vi "Main.vi"(11 "Module Admin":refnum<class "Delacor_lib_QMH_Module Admin.lvclass">) -> ()   [LabVIEW 2020, in "Logger.lvlib"]
doc: "This template is based off of the Queued Message Handler design pattern and the Queued Message Handler project template that ships with LabVIEW.\n\nThe main difference is that the queue is private to this module and communication between modules is performed via Broadcast and Request events.\n\nRequest events are wrapped in public API methods and are handled in the Event Handling Loop (EHL) of this VI. Any module can register for Broadcast events sent by this module. The EHL generates messages based on user interface actions.\n\nThe Message Handling Loop (MHL) processes messages generated by the EHL, or by other messages. The messages are string values, so new messages can be added easily to the Message Cases case structure in the MHL. Each message cluster can also provide an optional value for Message Data, which is a variant that can be converted to whatever message-specific data is required.\n_____\nBased on Delacor QMH Project Template 4.0.0.47.\n_____\nBased on DQMH Project Template 6.0.0.91."
uses:
  Logger.lvlib
  <vilib>/Delacor/Delacor QMH/Libraries/Module Admin_class/Delacor_lib_QMH_Module Admin.lvclass
  Module Data--cluster.ctl
  Stop Argument--cluster.ctl
  <vilib>/Delacor/Delacor QMH/Libraries/Message Queue_class/Delacor_lib_QMH_Message Queue.lvclass/Delacor_lib_QMH_Message Queue.ctl
  <vilib>/Delacor/Delacor QMH/Libraries/Module Admin_class/Delacor_lib_QMH_Module Admin.lvclass/Delacor_lib_QMH_Module Admin.ctl
  Initialize File Argument--cluster.ctl
  Initialize File (Reply Payload)--cluster.ctl
  Log Data Argument--cluster.ctl
  Stop Logging Argument--cluster.ctl
  Settings Editor/Update Application Settings (Reply Payload)--cluster.ctl
  Settings Editor/Settings--cluster.ctl
  CML Shared/Signal Type--enum.ctl
  CML Shared/Calibration Values--cluster.ctl
  <vilib>/Utility/miscctls.llb/LVPointTypeDef.ctl
  <vilib>/Delacor/Delacor QMH/Libraries/Message Queue_class/Delacor_lib_QMH_Enqueue Message (Single).vi
  <vilib>/Delacor/Delacor QMH/Libraries/Module Admin_class/Delacor_lib_QMH_Get External Launch.vi
  <vilib>/Utility/error.llb/Error Cluster From Error Code.vi
  <vilib>/ErrorRing/Error Ring.xnode
  <vilib>/Delacor/Delacor QMH/Libraries/Message Queue_class/Delacor_lib_QMH_Message Queue.lvclass
  Settings Editor/Settings Editor.lvlib
  CML Shared/CML Shared.lvlib
panel:
  out "Settings":T1
  out "error out":errorcluster
  # "This is a headless module. Show its panel to confirm that the Settings are updated correctly and other debugging tasks. Use the Settings Editor to change the settings for this module."
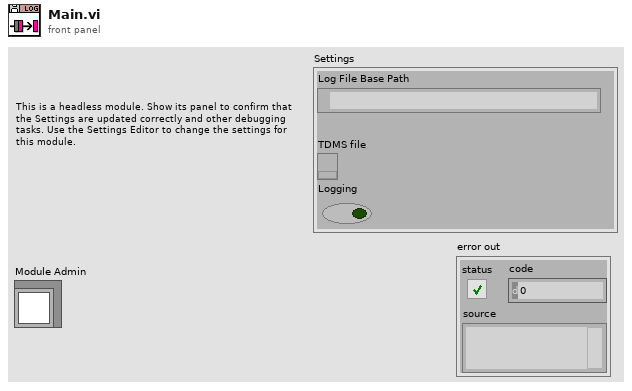
[diagram p1: front panel]
types:
  T1 = typedef "Logger.lvlib/Module Data--cluster.ctl" = cluster{"Log File Base Path":path, "TDMS file":refnum<k34>, "Logging":bool}
  T2 = typedef "Settings Editor.lvlib/Broadcast Events--cluster.ctl" = cluster{"Module Did Init":refnum<user-event>, "Status Updated":refnum<user-event>, "Error Reported":refnum<user-event>, "Module Did Stop":refnum<user-event>, "Update Module Execution Status":refnum<user-event>, "Application Settings Updated":refnum<user-event>}
  T3 = typedef "Logger.lvlib/Request Events--cluster.ctl" = cluster{"Stop Module":refnum<user-event>, "Show Panel":refnum<user-event>, "Hide Panel":refnum<user-event>, "Get Module Execution Status":refnum<user-event>, "Show Diagram":refnum<user-event>, "Stop Logging":refnum<user-event>, "Log Data":refnum<user-event>, "Initialize File":refnum<user-event>}
  T4 = enum32{"invalid lock state", "Not Locked", "Locked (No Password)", "Password-protected"}
  T5 = typedef "Logger.lvlib/Stop Argument--cluster.ctl" = cluster{"Origin":string, "Exit via Stop Module Req?":bool, "Wait for Module to stop?":bool}
  T6 = typedef "Logger.lvlib/Initialize File Argument--cluster.ctl" = cluster{"Wait Notifier":refnum<notifier>, "wait for reply":bool}
  T7 = typedef "Logger.lvlib/Log Data Argument--cluster.ctl" = cluster{"Waveforms":waveform(dbl)[]}
  T8 = typedef "Logger.lvlib/Stop Logging Argument--cluster.ctl" = cluster{"Boolean":bool}
  T9 = typedef "Settings Editor.lvlib/Update Application Settings (Reply Payload)--cluster.ctl" = cluster{"Settings":T10, "Update Settings_error":errorcluster}
  T10 = typedef "Settings Editor.lvlib/Settings--cluster.ctl" = cluster{"Signal Type":T11, "Calibration Array":T12[], "Log File Base Path":path}
  T11 = typedef "CML Shared.lvlib/Signal Type--enum.ctl" = enum16{"Sine Wave", "Square with Noise"}
  T12 = typedef "CML Shared.lvlib/Calibration Values--cluster.ctl" = cluster{"Slope":dbl, "Offset":dbl}
  T13 = typedef "LVPointTypeDef.ctl" = cluster{"Horizontal":i16, "Vertical":i16}
  T14 = enum32{"Invalid", "Standard", "Closed", "Hidden", "Minimized", "Maximized"}
  T15 = typedef "Logger.lvlib/Initialize File (Reply Payload)--cluster.ctl" = cluster{"File Path":path, "Initialize File_error":errorcluster}
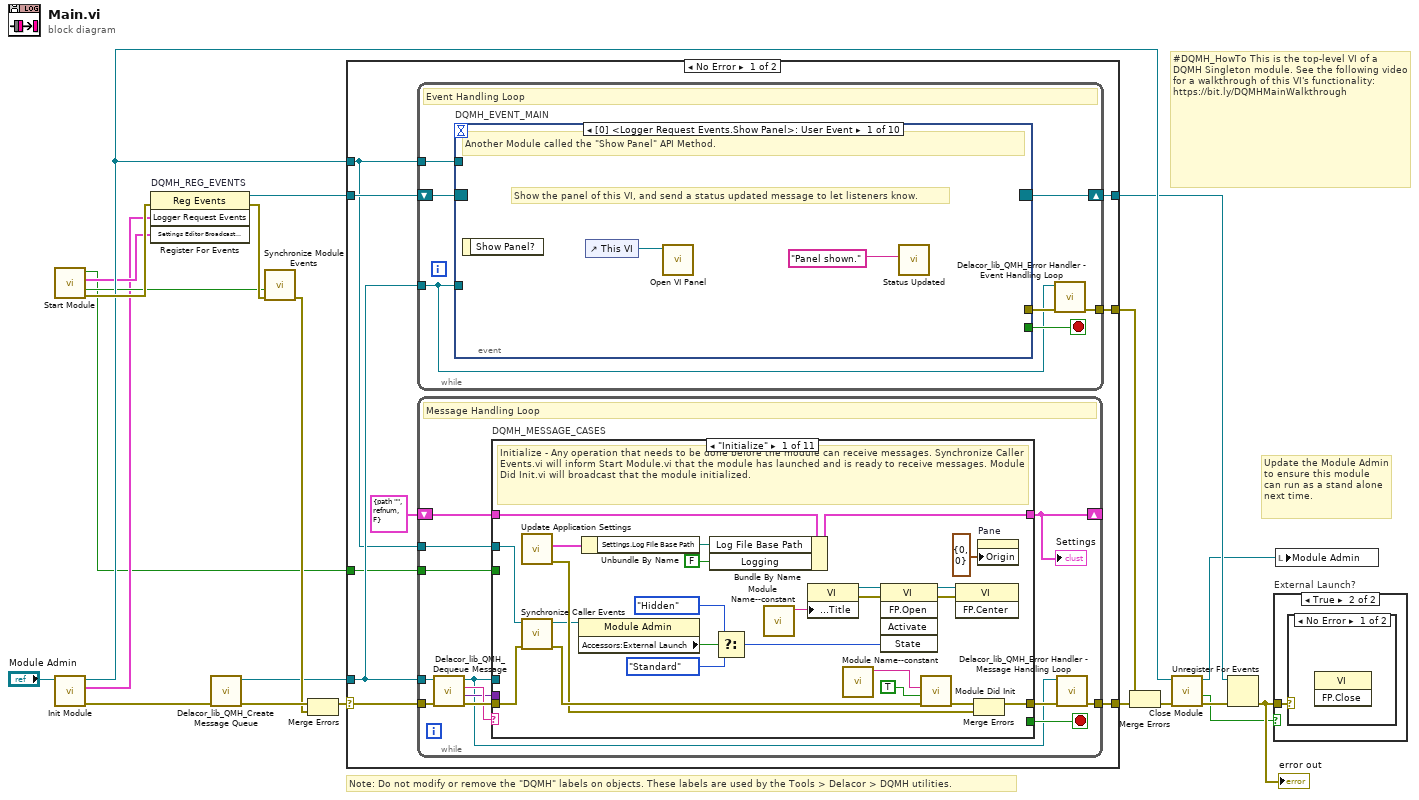
[diagram p0: block diagram]
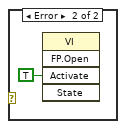
[diagram p3: hidden frame]
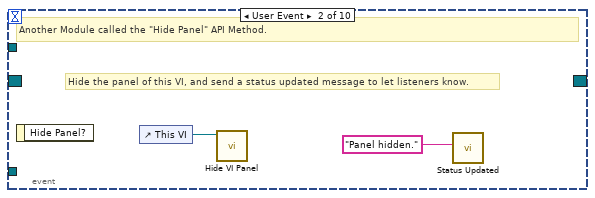
[diagram p4: hidden frame]
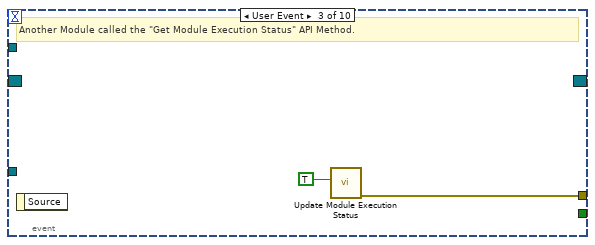
[diagram p5: hidden frame]
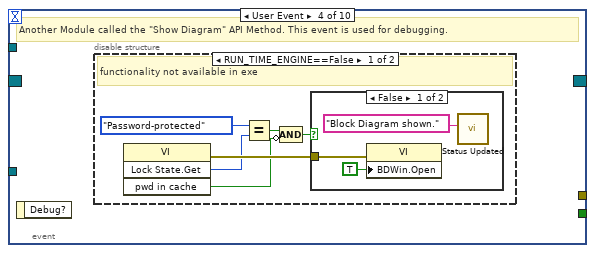
[diagram p6: hidden frame]
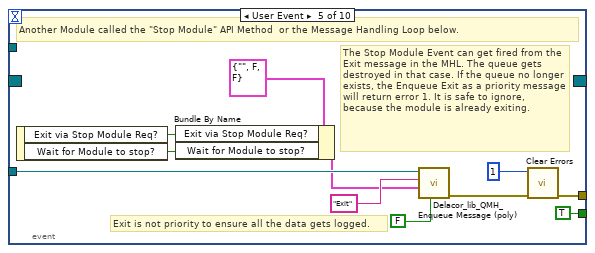
[diagram p9: hidden frame]
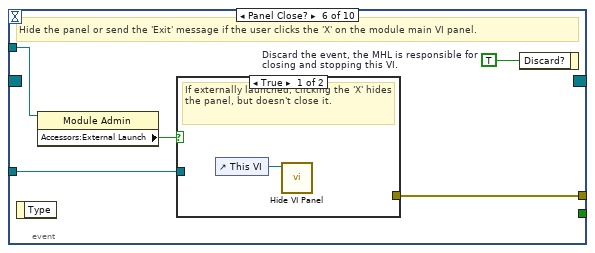
[diagram p10: hidden frame]
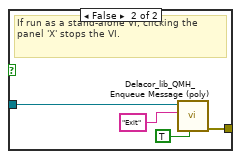
[diagram p11: hidden frame]
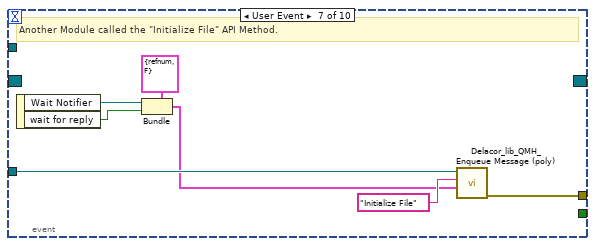
[diagram p12: hidden frame]
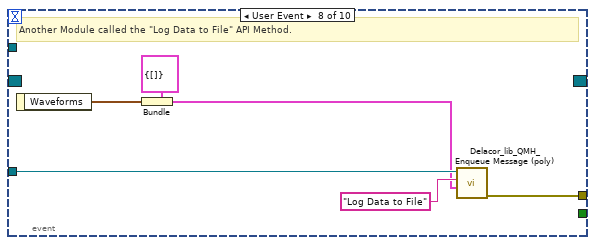
[diagram p13: hidden frame]
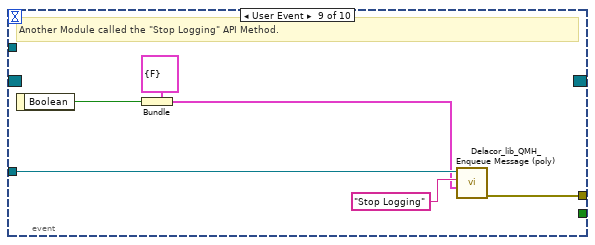
[diagram p14: hidden frame]
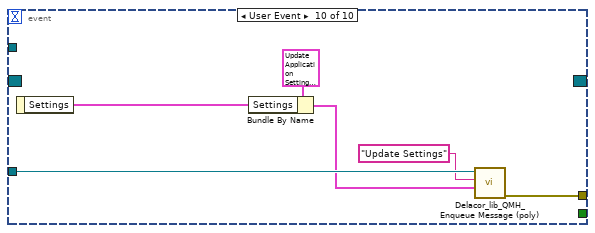
[diagram p15: hidden frame]
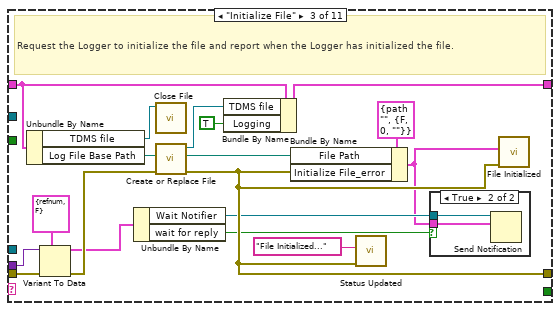
[diagram p17: hidden frame]
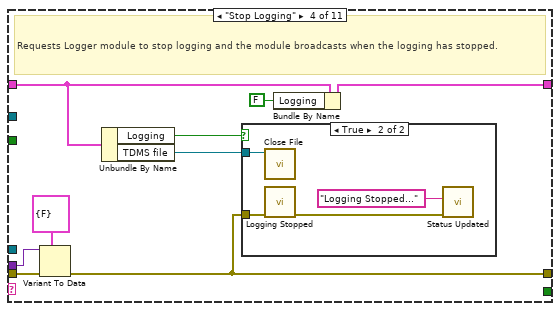
[diagram p19: hidden frame]
diagram:
  # "#DQMH_HowTo This is the top-level VI of a DQMH Singleton module. See the following video for a walkthrough of this VI's functionality: https://bit.ly/DQMHMainWalkthrough"
  # "Note: Do not modify or remove the \"DQMH\" labels on objects. These labels are used by the Tools > Delacor > DQMH utilities."
  # "Update the Module Admin to ensure this module can run as a stand alone next time."
  n1 = call "Start Module.vi"() -> ("error out"=w14:errorcluster, "Wait for Event Sync?"=w4:bool, "Settings Editor Broadcast Events"=w3:T2, "Module Was Already Running?"=w1:bool)  [unwired: 8 in]
  n2 = call "Init Module.vi"("Singleton Module Admin in"="Module Admin") -> ("error out"=w21:errorcluster, "Logger Request Events"=w2:T3, "Singleton Module Admin out"=w11:refnum<class "Delacor_lib_QMH_Module Admin.lvclass">)  [unwired: 8 in]
  n3 = register-events "DQMH_REG_EVENTS"(error in=w14, w2, w3) -> (reference out=w9:refnum<event-registration>, error out=w13:errorcluster)  [unwired: 1 in]
  n4 = call <vilib>:"Delacor_lib_QMH_Create Message Queue.vi"("error in"=w21) -> ("error out"=w16:errorcluster, "Message Queue"=w8:refnum<class "Delacor_lib_QMH_Message Queue.lvclass">)  [unwired: 9 in]
  n5 = call "Synchronize Module Events.vi"("error in (no error)"=w13, "Wait for Event Sync?"=w4) -> ("error out"=w12:errorcluster)  [unwired: 9 in]
  n6 = Merge Errors(w16, w12) -> (w15:errorcluster)
  n7 = case shown="No Error" w15 {
    selector: w15 -> [w29 w251]
    tunnel: [w31 w250] -> w22
    tunnel: [w28 w258] -> w10
    tunnel: w9 -> [w26 w258]
    tunnel: w8 -> [w25 w252]
    tunnel: [w30 _] -> w19
    tunnel: w11 -> [w24 w254]
    tunnel: w1 -> [w23 w253]
    frame No Error {
      n8 = while {
        tunnel: w25 -> [w32]
        shift-right: [w35] -> w28
        shift-left: w26 -> [w36]
        tunnel: [w37] -> w30
        tunnel: w24 -> [w33]
        stop <- w34 stop-if-true
        # "Event Handling Loop"
        n9 = event "DQMH_EVENT_MAIN" shown="[0] <Logger Request Events.Show Panel>: User Event" {
          selector: w36 -> [_ _ _ _ _ _ _ _ _ _]
          dyn-events: [_ _ _ _ _ _ _ _ _ _] -> w35
          timeout: _ -> [_ _ _ _ _ _ _ _ _ _]
          tunnel: [_ _ _ _ TRUE ("Discard?") _ _ _ _ _] -> w34
          tunnel: w32 -> [_ _ _ _ w60 w67 w80 w86 w92 w98]
          tunnel: [_ _ w44 _ w63 w69 w81 w87 w93 w99] -> w38
          tunnel: w33 -> [_ _ _ _ _ w66 _ _ _ _]
          event User Event {
            # "Show the panel of this VI, and send a status updated message to let listeners know."
            # "Another Module called the \"Show Panel\" API Method."
            n10 = event-data() -> ()  [unwired: 1 in, 1 out]
            n11 = control-ref of="This VI"() -> (w40:refnum<vi>)
            n12 = call "Open VI Panel.vi"("VI"=w40) -> ()  [unwired: 10 in, 1 out]
            n13 = call "Status Updated.vi"("Status"="Panel shown." ("format string")) -> ()  [unwired: 10 in, 1 out]
          }
          event User Event {
            # "Hide the panel of this VI, and send a status updated message to let listeners know."
            # "Another Module called the \"Hide Panel\" API Method."
            n14 = event-data() -> ()  [unwired: 1 in, 1 out]
            n15 = control-ref of="This VI"() -> (w42:refnum<vi>)
            n16 = call "Hide VI Panel.vi"("VI"=w42) -> ()  [unwired: 10 in, 1 out]
            n17 = call "Status Updated.vi"("Status"="Panel hidden." ("format string")) -> ()  [unwired: 10 in, 1 out]
          }
          event User Event {
            # "Another Module called the \"Get Module Execution Status\" API Method."
            n18 = event-data() -> ()  [unwired: 1 in, 1 out]
            n19 = call "Update Module Execution Status.vi"("Running?"=TRUE) -> ("error out"=w44:errorcluster)  [unwired: 10 in]
          }
          event User Event {
            # "Another Module called the \"Show Diagram\" API Method. This event is used for debugging."
            n20 = event-data() -> ()  [unwired: 1 in, 1 out]
            n21 = disable-structure shown="RUN_TIME_ENGINE==False" {
              frame condition #0 (active) {
                # "functionality not available in exe"
                n22 = invoke class="VI" method="Lock State.Get"() -> (error out=w50:errorcluster, "Get Lock State"=w49:T4, "pwd in cache"=w46:bool)  [unwired: 4 in, 1 out]
                n23 = Equal?(x=T4."Password-protected", y=w49) -> (x = y?=w47:bool)
                n24 = Compound Arithmetic op=AND(w47, invert w46) -> (w45:bool)
                n25 = case shown="False" w45 {
                  tunnel: w50 -> [w53 _]
                  frame False {
                    n26 = property class="VI"(error in=w53, "BDWin.Open"=TRUE ("Block Diagram Window:Open")) -> ()  [unwired: 1 in, 2 out]
                    n27 = call "Status Updated.vi"("Status"="Block Diagram shown." ("format string")) -> ()  [unwired: 10 in, 1 out]
                  }
                  frame True {
                    # "Password-protected VI, and the password is not in the cache. Do not show the diagram."
                  }
                }
              }
              frame condition #1 {
              }
            }
          }
          event User Event {
            # "Exit is not priority to ensure all the data gets logged."
            # "The Stop Module Event can get fired from the Exit message in the MHL. The queue gets destroyed in that case. If the queue no longer exists, the Enqueue Exit as a priority message will return error 1. It is safe to ignore, because the module is already exiting."
            # "Another Module called the \"Stop Module\" API Method  or the Message Handling Loop below."
            n28 = event-data() -> ("Exit via Stop Module Req?"=w56:bool, "Wait for Module to stop?"=w55:bool)  [unwired: 1 in]
            n29 = Bundle By Name(cluster=T5 {"Origin"="", "Exit via Stop Module Req?"=FALSE, "Wait for Module to stop?"=FALSE} ("Stop Argument"), "Exit via Stop Module Req?"=w56, "Wait for Module to stop?"=w55) -> (w54:T5)
            n30 = call-poly <vilib>:"Delacor_lib_QMH_Enqueue Message (poly).vi"("Priority Message? (F)"=FALSE, "Message Data"=w54, "Message"="Exit", "Message Queue in"=w60) -> ("error out"=w64:errorcluster)  [unwired: 6 in, 1 out]
            n31 = call <vilib>:"Clear Errors.vi"("error in (no error)"=w64, "specific error code to clear (0: all)"=1) -> ("error out"=w63:errorcluster)  [unwired: 4 in, 1 out]
          }
          event Panel Close? {
            w68 = TRUE  # Discard the event, the MHL is responsible for closing and stopping this VI.
            # "Hide the panel or send the 'Exit' message if the user clicks the 'X' on the module main VI panel."
            n32 = event-data() -> ()  [unwired: 1 in, 1 out]
            n33 = property class="Module Admin"(reference=w66) -> ("Accessors:External Launch"=w65:bool)  [unwired: 1 in, 2 out]
            n34 = case shown="True" w65 {
              tunnel: w67 -> [_ w73]
              tunnel: [_ w74] -> w69
              frame True {
                # "If externally launched, clicking the 'X' hides the panel, but doesn't close it."
                n35 = control-ref of="This VI"() -> (w70:refnum<vi>)
                n36 = call "Hide VI Panel.vi"("VI"=w70) -> ()  [unwired: 10 in, 1 out]
              }
              frame False {
                # "If run as a stand-alone VI, clicking the panel 'X' stops the VI."
                n37 = call-poly <vilib>:"Delacor_lib_QMH_Enqueue Message (poly).vi"("Priority Message? (F)"=TRUE, "Message"="Exit", "Message Queue in"=w73) -> ("error out"=w74:errorcluster)  [unwired: 7 in, 1 out]
              }
            }
            n38 = event-data("Discard?"=w68) -> ()  [unwired: 1 in, 1 out]
          }
          event User Event {
            # "Another Module called the \"Initialize File\" API Method."
            n39 = event-data() -> ("Wait Notifier"=w76:refnum<notifier>, "wait for reply"=w75:bool)  [unwired: 1 in]
            n40 = Bundle(cluster=T6 {"Wait Notifier"=refnum, "wait for reply"=FALSE} ("Initialize File Argument"), "Wait Notifier"=w76, "wait for reply"=w75) -> (w77:T6)
            n41 = call-poly <vilib>:"Delacor_lib_QMH_Enqueue Message (poly).vi"("Message Data"=w77, "Message"="Initialize File", "Message Queue in"=w80) -> ("error out"=w81:errorcluster)  [unwired: 7 in, 1 out]
          }
          event User Event {
            # "Another Module called the \"Log Data to File\" API Method."
            n42 = event-data() -> ("Waveforms"=w82:waveform(dbl)[])  [unwired: 1 in]
            n43 = Bundle(cluster=T7 {"Waveforms"=[]} ("Log Data to File Argument"), "Waveforms"=w82) -> (w83:T7)
            n44 = call-poly <vilib>:"Delacor_lib_QMH_Enqueue Message (poly).vi"("Message Data"=w83, "Message"="Log Data to File", "Message Queue in"=w86) -> ("error out"=w87:errorcluster)  [unwired: 7 in, 1 out]
          }
          event User Event {
            # "Another Module called the \"Stop Logging\" API Method."
            n45 = event-data() -> ("Boolean"=w88:bool)  [unwired: 1 in]
            n46 = Bundle(cluster=T8 {"Boolean"=FALSE} ("Stop Logging Argument"), "Boolean"=w88) -> (w89:T8)
            n47 = call-poly <vilib>:"Delacor_lib_QMH_Enqueue Message (poly).vi"("Message Data"=w89, "Message"="Stop Logging", "Message Queue in"=w92) -> ("error out"=w93:errorcluster)  [unwired: 7 in, 1 out]
          }
          event User Event {
            n48 = event-data() -> ("Settings"=w95:T10)  [unwired: 1 in]
            n49 = Bundle By Name(cluster=T9 {"Settings"={"Signal Type"=enum."Sine Wave", "Calibration Array"=[], "Log File Base Path"=path ""}, "Update Settings_error"={"status"=FALSE, "code"=0, "source"=""}} ("Settings Updated Argument"), "Settings"=w95) -> (w94:T9)
            n50 = call-poly <vilib>:"Delacor_lib_QMH_Enqueue Message (poly).vi"("Message Data"=w94, "Message"="Update Settings", "Message Queue in"=w98) -> ("error out"=w99:errorcluster)  [unwired: 7 in, 1 out]
          }
        }
        n51 = call-dynamic "Delacor_lib_QMH_Error Handler - Event Handling Loop.vi"("error in"=w38, "Message Queue in"=w32) -> ("dup error in"=w37:errorcluster)  [unwired: 8 in, 1 out]
      }
      n52 = while {
        tunnel: w25 -> [w103]
        shift-right: [w107] -> _
        shift-left: T1 {"Log File Base Path"=path "", "TDMS file"=refnum, "Logging"=FALSE} ("Data Cluster") -> [w108]
        tunnel: w29 -> [w111]
        tunnel: [w109] -> w31
        tunnel: w24 -> [w101]
        tunnel: w23 -> [w100]
        stop <- w106 stop-if-true
        # "Message Handling Loop"
        n53 = call-dynamic "Delacor_lib_QMH_Dequeue Message.vi"("error in"=w111, "Message Queue in"=w103) -> ("error out"=w110:errorcluster, "Message Data"=w104:variant, "Message"=w105:string, "Message Queue out"=w102:refnum<class "Delacor_lib_QMH_Message Queue.lvclass">)  [unwired: 6 in]
        n54 = case "DQMH_MESSAGE_CASES" shown="\"Initialize\"" w105 {
          selector: w105 -> [_ _ _ _ _ _ _ _ _ _ w237]
          tunnel: w102 -> [_ _ _ _ _ _ _ _ w203 w227 _]
          tunnel: w110 -> [w134 w138 w155 w167 w180 w190 w198 w200 w210 w233 w239]
          tunnel: [w131 w138 w156 w166 w173 w188 w197 w200 w206 w230 w240] -> w112
          tunnel: w108 -> [w121 w137 w144 w163 w179 w183 w196 w199 w205 w219 w238]
          tunnel: [w115 w137 w143 w160 w177 w183 w196 w199 w205 w219 w238] -> w107
          tunnel: [_ _ _ _ _ _ _ _ _ w226 _] -> w106
          tunnel: w104 -> [_ _ w153 w165 w178 w187 _ _ w204 w225 _]
          tunnel: w101 -> [w122 _ _ _ _ _ _ _ w202 w220 _]
          tunnel: w100 -> [_ _ _ _ _ _ _ _ _ w217 _]
          frame "Initialize" {
            # "Initialize - Any operation that needs to be done before the module can receive messages. Synchronize Caller Events.vi will inform Start Module.vi that the module has launched and is ready to receive messages. Module Did Init.vi will broadcast that the module initialized."
            n55 = call "Update Application Settings.vi"() -> ("error out"=w130:errorcluster, "Reply Payload"=w116:T9)  [unwired: 9 in, 1 out]
            n56 = call "Synchronize Caller Events.vi"("error in (no error)"=w134, "Singleton Module Admin in"=w122) -> ("error out"=w133:errorcluster, "Singleton Module Admin out"=w118:refnum<class "Delacor_lib_QMH_Module Admin.lvclass">)  [unwired: 8 in]
            n57 = property class="Module Admin"(reference=w118) -> ("Accessors:External Launch"=w126:bool)  [unwired: 1 in, 2 out]
            n58 = Unbundle By Name(w116) -> ("Settings.Log File Base Path"=w114:path)
            n59 = Bundle By Name(cluster=w121, "Log File Base Path"=w114, "Logging"=FALSE) -> (w115:T1)
            n60 = Select(t=T14."Hidden" ("State"), s=w126, f=T14."Standard" ("State")) -> (s? t:f=w123:T14)
            n61 = call "Module Name--constant.vi"() -> ("Module Name"=w129:string)  [unwired: 11 in]
            n62 = property class="VI"("Front Panel.Title"=w129) -> (reference out=w128:refnum<vi>, error out=w136:errorcluster)  [unwired: 2 in]
            n63 = call "Module Name--constant.vi"() -> ("Module Name"=w119:string)  [unwired: 11 in]
            n64 = invoke class="VI" method="FP.Open"(reference=w128, error in=w136, "State"=w123) -> (reference out=w127:refnum<vi>, error out=w135:errorcluster)  [unwired: 2 in, 3 out]
            n65 = call "Module Did Init.vi"("error in (no error)"=w133, "Initialized?"=TRUE, "Origin"=w119) -> ("error out"=w132:errorcluster)  [unwired: 8 in]
            n66 = invoke class="VI" method="FP.Center"(reference=w127, error in=w135) -> ()  [unwired: 1 in, 3 out]
            n67 = Merge Errors(w132, w130) -> (w131:errorcluster)
            n68 = property on="Pane" class="Pane"("Origin"=T13 {"Horizontal"=0, "Vertical"=0}) -> ()  [unwired: 2 in, 2 out]
          }
          frame "---Module Specific---" {
            # "Separator -- The following cases handle messages specific to this Module."
          }
          frame "Initialize File" {
            # "Request the Logger to initialize the file and report when the Logger has initialized the file."
            n69 = Unbundle By Name(w144) -> ("TDMS file"=w139:refnum<k34>, "Log File Base Path"=w146:path)
            n70 = Variant To Data(error in=w155, type=T6 {"Wait Notifier"=refnum, "wait for reply"=FALSE} ("Initialize File Argument"), Variant=w153) -> (data=w151:T6, error out=w154:errorcluster)
            n71 = Unbundle By Name(w151) -> ("Wait Notifier"=w150:refnum<notifier>, "wait for reply"=w149:bool)
            n72 = call "Close File.vi"("Refnum out"=w139) -> ()  [unwired: 10 in, 1 out]
            n73 = call "Create or Replace File.vi"("error in (no error)"=w154, "Log File Base Path"=w146) -> ("error out"=w156:errorcluster, "File Path"=w142:path, "Refnum out"=w145:refnum<k34>)  [unwired: 7 in]
            n74 = Bundle By Name(cluster=w144, "TDMS file"=w145, "Logging"=TRUE) -> (w143:T1)
            n75 = Bundle By Name(cluster=T15 {"File Path"=path "", "Initialize File_error"={"status"=FALSE, "code"=0, "source"=""}} ("Initialize File (Reply Payload)"), "File Path"=w142, "Initialize File_error"=w156) -> (w147:T15)
            n76 = call "Status Updated.vi"("error in (no error)"=w156, "Status"="File Initialized...") -> ()  [unwired: 9 in, 1 out]
            n77 = case shown="True" w149 {
              tunnel: w150 -> [_ w158]
              tunnel: w147 -> [_ w157]
              frame False {
              }
              frame True {
                n78 = Send Notification(notification=w157, notifier=w158) -> ()  [unwired: 1 in, 2 out]
              }
            }
            n79 = call "File Initialized.vi"("error in (no error)"=w156, "Reply Payload"=w147) -> ()  [unwired: 9 in, 1 out]
          }
          frame "Stop Logging" {
            # "Requests Logger module to stop logging and the module broadcasts when the logging has stopped."
            n80 = Variant To Data(error in=w167, type=T8 {"Boolean"=FALSE} ("Stop Logging Argument"), Variant=w165) -> (error out=w166:errorcluster)  [unwired: 1 out]
            n81 = Unbundle By Name(w163) -> ("Logging"=w162:bool, "TDMS file"=w161:refnum<k34>)
            n82 = case shown="True" w162 {
              tunnel: w166 -> [_ w171]
              tunnel: w161 -> [_ w168]
              frame False {
                # "We were not logging, so this is a no-op."
              }
              frame True {
                n83 = call "Close File.vi"("Refnum out"=w168) -> ()  [unwired: 10 in, 1 out]
                n84 = call "Logging Stopped.vi"("error in (no error)"=w171) -> ("error out"=w170:errorcluster)  [unwired: 10 in]
                n85 = call "Status Updated.vi"("error in (no error)"=w170, "Status"="Logging Stopped...") -> ()  [unwired: 9 in, 1 out]
              }
            }
            n86 = Bundle By Name(cluster=w163, "Logging"=FALSE) -> (w160:T1)
          }
          frame "Update Settings" {
            n87 = Variant To Data(error in=w180, type=T9 {"Settings"={"Signal Type"=enum."Sine Wave", "Calibration Array"=[], "Log File Base Path"=path ""}, "Update Settings_error"={"status"=FALSE, "code"=0, "source"=""}} ("Settings Updated Argument"), Variant=w178) -> (data=w176:T9, error out=w173:errorcluster)
            n88 = Unbundle By Name(w176) -> ("Settings.Log File Base Path"=w175:path)
            n89 = Bundle By Name(cluster=w179, "Log File Base Path"=w175) -> (w177:T1)
            n90 = call "Status Updated.vi"("error in (no error)"=w173, "Status"="Settings Updated") -> ()  [unwired: 9 in, 1 out]
          }
          frame "Log Data to File" {
            # "Requests Logger module to log data to file"
            n91 = Variant To Data(error in=w190, type=T7 {"Waveforms"=[]} ("Log Data to File Argument"), Variant=w187) -> (data=w185:T7, error out=w189:errorcluster)
            n92 = Unbundle By Name(w183) -> ("Logging"=w181:bool, "TDMS file"=w182:refnum<k34>)
            n93 = Unbundle By Name(w185) -> ("Waveforms"=w184:waveform(dbl)[])
            n94 = case shown="False" w181 {
              tunnel: w189 -> [w191 w195]
              tunnel: [w191 w194] -> w188
              tunnel: w184 -> [_ w193]
              tunnel: w182 -> [_ w192]
              frame False {
                # "We are not currently logging, so this action is a no-op."
              }
              frame True {
                n95 = call "Log Data to File.vi"("error in (no error)"=w195, "Data to log"=w193, "TDMS File Reference"=w192) -> ("error out"=w194:errorcluster)  [unwired: 8 in]
              }
            }
          }
          frame "---Copy This Frame---" {
            # "Duplicate this frame when creating new messages.  Change this comment in the duplicated frame to describe this message."
            n96 = Merge Errors(w198) -> (w197:errorcluster)
          }
          frame "---Exit and Error Handling---" {
            # "Separator - The following cases handle errors and exit messages."
          }
          frame "Error" {
            # "Error - Check the error message data and respond accordingly. This message is sent by the \"Error Handler\" VIs at the end of each loop in this application."
            n97 = property class="Module Admin"(reference=w202) -> ("Accessors:External Launch"=w201:bool)  [unwired: 1 in, 2 out]
            n98 = Variant To Data(error in=w210, type=errorcluster {"status"=FALSE, "code"=0, "source"=""} ("error constant"), Variant=w204) -> (data=w211:errorcluster, error out=w208:errorcluster)
            n99 = call "Error Reported.vi"("Error"=w211) -> ()  [unwired: 10 in, 1 out]
            n100 = case shown="False" w201 {
              tunnel: [w216 _] -> w207
              tunnel: w203 -> [w214 _]
              tunnel: w211 -> [w215 _]
              frame False {
                # "If the module is running standalone, then pop up an error dialog and call the \"Exit\" message."
                n101 = call <vilib>:"Simple Error Handler.vi"("error in (no error)"=w215) -> ()  [unwired: 4 in, 5 out]
                n102 = call-poly <vilib>:"Delacor_lib_QMH_Enqueue Message (poly).vi"("Priority Message? (F)"=TRUE, "Message"="Exit", "Message Queue in"=w214) -> ("error out"=w216:errorcluster)  [unwired: 7 in, 1 out]
              }
              frame True {
                # "If the module was launched externally, calling the Error Reported broadcast VI is the only action performed by the \"Error\" message. The module's caller can then process the error appropriately."
              }
            }
            n103 = Merge Errors(w208, w207) -> (w206:errorcluster)
            n104 = local write "error out"(w206) -> ()
          }
          frame "Exit" {
            w224 = 91  # 91: not all Exit messages will have an argument
            w226 = TRUE  # Stop the VI
            # "Release the message queue reference"
            # "Exit - Exit the application."
            n105 = Variant To Data(error in=w233, type=T5 {"Origin"="", "Exit via Stop Module Req?"=FALSE, "Wait for Module to stop?"=FALSE} ("Stop Argument"), Variant=w225) -> (data=w222:T5, error out=w229:errorcluster)
            n106 = call <vilib>:"Clear Errors.vi"("error in (no error)"=w229, "specific error code to clear (0: all)"=w224) -> ("error out"=w232:errorcluster)  [unwired: 4 in, 1 out]
            n107 = Unbundle By Name(w219) -> ("TDMS file"=w218:refnum<k34>)
            n108 = control-ref of="This VI"() -> (w221:refnum<vi>)
            n109 = call-dynamic "Delacor_lib_QMH_Release Message Queue.vi"("error in"=w232, "Message Queue"=w227) -> ("error out"=w231:errorcluster)  [unwired: 9 in]
            n110 = call "Handle Exit.vi"("Stop Argument"=w222, "Admin in"=w220, "VI reference"=w221) -> ("error out"=w228:errorcluster)  [unwired: 7 in, 1 out]
            n111 = call "Close File.vi"("Refnum out"=w218) -> ()  [unwired: 10 in, 1 out]
            n112 = case "Settings Editor was\nalready running?" shown="False" w217 {
              frame False {
                n113 = call "Module Name--constant.vi"() -> ("Module Name"=w235:string)  [unwired: 11 in]
                n114 = call "Stop Module.vi"("Wait for Module to Stop? (F)"=TRUE, "Origin"=w235) -> ()  [unwired: 9 in, 1 out]
              }
              frame True {
                # "Another Module is\nin charge of stopping Settings Editor"
              }
            }
            n115 = Merge Errors(w231, w228) -> (w230:errorcluster)
          }
          frame Default {
            # "'Default' case only runs if there is a message that isn't defined in any of the other cases.  Output a programming error."
            n116 = call "Module Name--constant.vi"() -> ("Module Name"=w236:string)  [unwired: 11 in]
            n117 = xnode "Error Ring"("parameter 0"=w237, "parameter 1"=w236) -> ("error out"=w241:errorcluster)
            n118 = Merge Errors(w239, w241) -> (w240:errorcluster)
          }
        }
        "Settings" <- w107
        n119 = call-dynamic "Delacor_lib_QMH_Error Handler - Message Handling Loop.vi"("error in"=w112, "Message Queue in"=w102) -> ("dup error in"=w109:errorcluster)  [unwired: 8 in, 1 out]
      }
    }
    frame Error {
      # "Synchronize Caller Events.vi will inform Start Module.vi that the module has launched and will let the code calling Start Module.vi register for broadcasts and would permit the caller receive the broadcast that an error occurred at launch time."
      n120 = call "Synchronize Caller Events.vi"("Singleton Module Admin in"=w254) -> ("error out"=w259:errorcluster)  [unwired: 9 in, 1 out]
      n121 = call-dynamic "Delacor_lib_QMH_Release Message Queue.vi"("error in"=w251, "Message Queue"=w252) -> ("error out"=w250:errorcluster)  [unwired: 9 in]
      n122 = call "Module Name--constant.vi"() -> ("Module Name"=w257:string)  [unwired: 11 in]
      n123 = case "Settings Editor was\nalready running?" shown="False" w253 {
        frame False {
          n124 = call "Module Name--constant.vi"() -> ("Module Name"=w262:string)  [unwired: 11 in]
          n125 = call "Stop Module.vi"("Wait for Module to Stop? (F)"=TRUE, "Origin"=w262) -> ()  [unwired: 9 in, 1 out]
        }
        frame True {
          # "Another Module is\nin charge of stopping Settings Editor"
        }
      }
      n126 = Format Into String(format string="An error occurred during initialization. %s is no longer running.", w257) -> (resulting string=w255:string)  [unwired: 2 in, 1 out]
      n127 = Merge Errors(w251, w259) -> (w260:errorcluster)
      n128 = call "Error Reported.vi"("Additional Information"=w255, "Error"=w260) -> ()  [unwired: 9 in, 1 out]
    }
  }
  n129 = Merge Errors(w19, w22) -> (w18:errorcluster)
  n130 = call "Close Module.vi"("error in (no error)"=w18, "Module Admin in"=w11) -> ("error out"=w20:errorcluster, "External Launch"=w5:bool, "Module Admin out"=w6:refnum<class "Delacor_lib_QMH_Module Admin.lvclass">)  [unwired: 7 in]
  n131 = Unregister For Events(event registration refnum=w10, error in=w20) -> (error out=w17:errorcluster)
  "error out" <- w17
  n132 = case "External Launch?" shown="True" w5 {
    tunnel: w17 -> [_ w263]
    frame False {
    }
    frame True {
      n133 = case shown="No Error" w263 {
        frame No Error {
          n134 = invoke class="VI" method="FP.Close"() -> ()  [unwired: 3 in, 3 out]
        }
        frame Error {
          n135 = invoke class="VI" method="FP.Open"("Activate"=TRUE ("Activate?")) -> ()  [unwired: 4 in, 5 out]
        }
      }
    }
  }
  n136 = local write "Module Admin"(w6) -> ()
